vi "Run All Tests.vi"(8 "error in":errorcluster) -> (0 "error out":errorcluster)   [LabVIEW 2020]
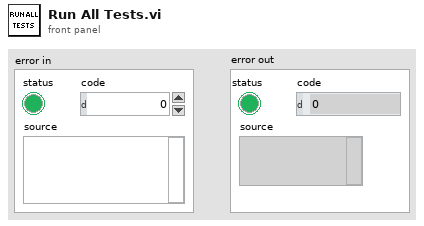
[diagram p1: front panel]
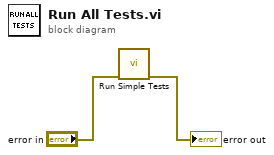
[diagram p0: block diagram]
diagram:
  n1 = call "Run Simple Tests.vi"("error in"="error in") -> ("error out"=→"error out":errorcluster)  [unwired: 10 in]
